vi "ActualizarTablacafe.vi"(8 "error in (no error)":errorcluster, 11 "coffee Actor in":refnum<class "coffee Actor.lvclass">) -> (0 "error out":errorcluster, 3 "coffee Actor out":refnum<class "coffee Actor.lvclass">)   [LabVIEW 2019, in "coffee Actor.lvlib" / "coffee Actor.lvclass"]
uses:
  coffee Actor.lvclass
  coffee Actor.lvclass/coffee Actor.ctl
  <vilib>/Utility/config.llb/Read Key (Double).vi
  <vilib>/Utility/config.llb/Read Key (String).vi
  <vilib>/Utility/config.llb/NI_LVConfig.lvlib
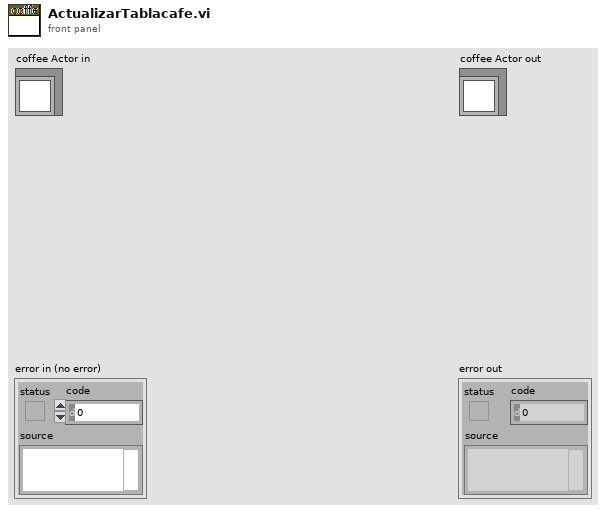
[diagram p1: front panel]
types:
  T1 = typedef "NI_LVConfig.lvlib/Config Data RefNum.ctl" = refnum<k1>
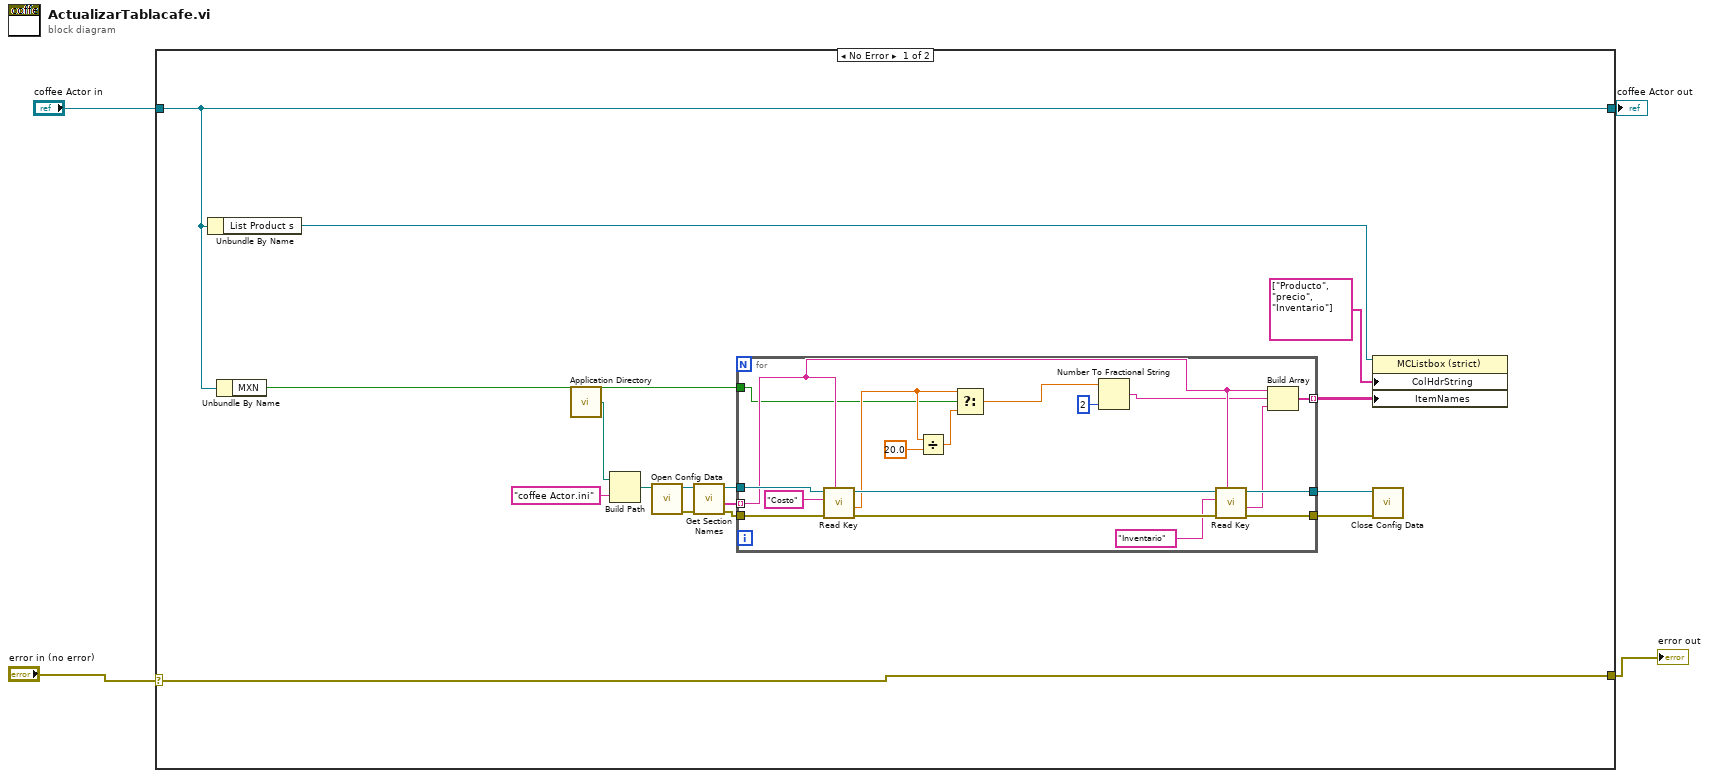
[diagram p0: block diagram]
diagram:
  n1 = case shown="No Error" "error in (no error)" {
    selector: "error in (no error)" -> [w20 w40]
    tunnel: [w20 w40] -> w3
    tunnel: [w6 w39] -> w1
    tunnel: "coffee Actor in" -> [w6 w39]
    frame No Error {
      n2 = Unbundle By Name(w6) -> ("List Product s"=w5:refnum<vi>)
      n3 = Unbundle By Name(w6) -> ("MXN"=w15:bool)
      n4 = call <vilib>:"Application Directory.vi"() -> ("Application Directory"=w19:path)
      n5 = Build Path(base path=w19, name or relative path="coffee Actor.ini") -> (appended path=w18:path)
      n6 = call <vilib>:"Open Config Data.vi"("configuration file path"=w18) -> ("error out"=w12:errorcluster, "refnum"=w13:T1)  [unwired: 8 in, 1 out]
      n7 = call <vilib>:"Get Section Names.vi"("error in (no error)"=w12, "refnum"=w13) -> ("error out"=w10:errorcluster, "section names"=w9:string[], "refnum out"=w11:T1)  [unwired: 7 in]
      n8 = for {
        tunnel: w10 -> [w37]
        tunnel: w11 -> [w38]
        tunnel: [w34] -> w16
        tunnel: [w33] -> w17
        tunnel: w15 -> [w21]
        tunnel: w9 -> [w30] mode=indexing
        tunnel: [w28] -> w8 mode=indexing
        n9 = call-poly <vilib>:"Read Key.vi"("section"=w30, "error in (no error)"=w37, "key"="Costo" ("section"), "refnum"=w38) -> ("error out"=w36:errorcluster, "value"=w24:dbl, "refnum out"=w35:T1)  [unwired: 4 in, 1 out]
        n10 = Divide(x=w24, y=20.0) -> (x/y=w22:dbl)
        n11 = Select(t=w24, s=w21, f=w22) -> (s? t:f=w25:dbl)
        n12 = Number To Fractional String(number=w25, precision (6)=i16 2) -> (F-format string=w27:string)  [unwired: 2 in]
        n13 = call-poly <vilib>:"Read Key.vi"("section"=w30, "error in (no error)"=w36, "key"="Inventario" ("section"), "refnum"=w35) -> ("error out"=w34:errorcluster, "value"=w29:string, "refnum out"=w33:T1)  [unwired: 4 in, 1 out]
        n14 = Build Array(w30, w27, w29) -> (w28:string[])
      }
      n15 = property class="MCListbox (strict)"(reference=w5, "ColHdrString"=string[] ["Producto", "precio", "Inventario"] ("Column Header Strings[]"), "ItemNames"=w8) -> ()  [unwired: 1 in, 2 out]
      n16 = call <vilib>:"Close Config Data.vi"("error in (no error)"=w16, "refnum"=w17) -> ()  [unwired: 8 in, 2 out]
    }
    frame Error {
    }
  }
  "error out" <- w3
  "coffee Actor out" <- w1
